vi "Initialize Channel Objects.vi"(8 "error in (no error)":errorcluster, 11 "Default Channel Status":bool) -> (0 "error out":errorcluster, 2 "Active Channel[]":bool[](array[boolean]), 3 "Channel Info[]":T1[](array[typedef]))   [LabVIEW 2020, in "Plugin.lvlib" / "Plugin_UI.lvclass"]
doc: "Creates the default channels."
uses:
  Plugin_UI.lvclass
  builds/Libraries/LabSys Framework.lvlibp/Configuration Storage/Test Configuration/Channel Information.ctl
  builds/Libraries/LabSys Framework.lvlibp/Configuration Storage/Test Configuration/Channel Directions.ctl
  builds/Libraries/LabSys Framework.lvlibp/Configuration Storage/Test Configuration/Scaling Information.ctl
  builds/Libraries/LabSys Framework.lvlibp/Configuration Storage/Test Configuration/Scaling Types.ctl
  builds/Libraries/Framework Base Library.lvlibp/Value Types.ctl
  builds/Libraries/LabSys Framework.lvlibp/Configuration Storage/Test Configuration/Subchannel Information.ctl
  Channels/Output Channels/Output Channels.lvclass
  C:/SVN_LabSys/labsys_lvcode/LabSys_SourceCode/Plugin Template/Source/Code/Channels/Plugin_Channels.lvclass
  Channels/Typedefs/Channel Type.ctl
  Channels/Input Channels/Input Channels.lvclass
  Channels/Plugin_Channels.lvclass
  builds/Libraries/LabSys Framework.lvlibp/Configuration Storage/Test Configuration/Test Configuration.lvclass
  builds/Libraries/Framework Base Library.lvlibp
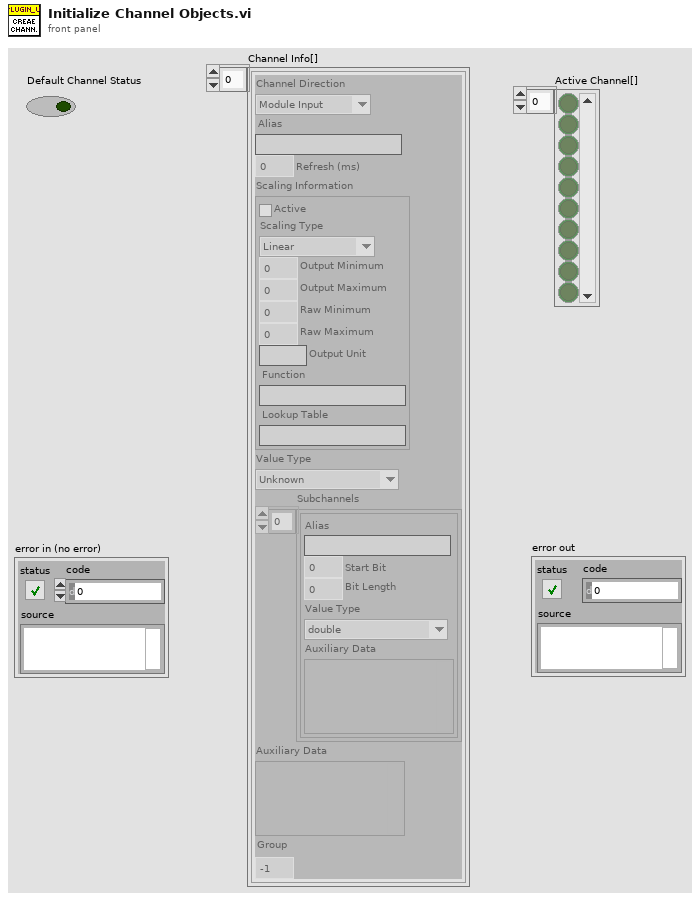
[diagram p1: front panel]
types:
  T1 = typedef "LabSys Framework.lvlibp/Configuration Storage.lvlib/Test Configuration.lvclass/Channel Information.ctl" = cluster{"Channel Direction":T2, "Alias":string, "Refresh (ms)":dbl, "Scaling Information":T3, "Value Type":T5, "Subchannels":T6[], "Auxiliary Data":variant, "Group":i32}
  T2 = typedef "LabSys Framework.lvlibp/Configuration Storage.lvlib/Test Configuration.lvclass/Channel Directions.ctl" = enum8{"Module Input", "Module Output"}
  T3 = typedef "LabSys Framework.lvlibp/Configuration Storage.lvlib/Test Configuration.lvclass/Scaling Information.ctl" = cluster{"Active":bool, "Scaling Type":T4, "Output Minimum":dbl, "Output Maximum":dbl, "Raw Minimum":dbl, "Raw Maximum":dbl, "Output Unit":string, "Function":string, "Lookup Table":string}
  T4 = typedef "LabSys Framework.lvlibp/Configuration Storage.lvlib/Test Configuration.lvclass/Scaling Types.ctl" = enum8{"Linear", "Function", "Lookup Table"}
  T5 = typedef "Framework Base Library.lvlibp/Value Types.ctl" = enum8{"Unknown", "double", "double array", "Waveform", "DigWaveform", "Boolean", "Decimal", "String", "Db2Message", "Byte Array", "Unsigned Decimal"}
  T6 = typedef "LabSys Framework.lvlibp/Configuration Storage.lvlib/Test Configuration.lvclass/Subchannel Information.ctl" = cluster{"Alias":string, "Start Bit":u32, "Bit Length":u32, "Value Type":T5, "Auxiliary Data":variant}
  T7 = typedef "Plugin.lvlib/Plugin_Channels.lvclass/Channel Type.ctl" = enum16{"Input", "Output"}
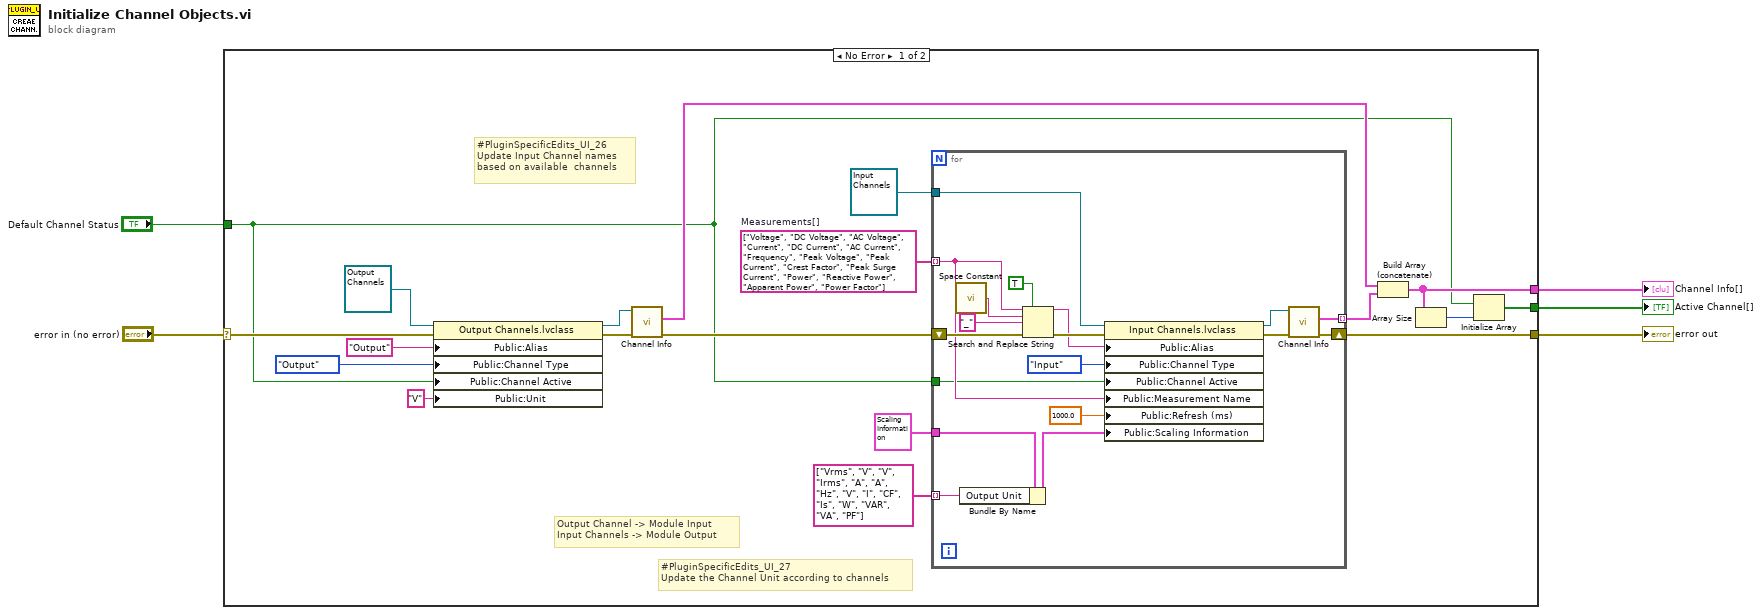
[diagram p0: block diagram]
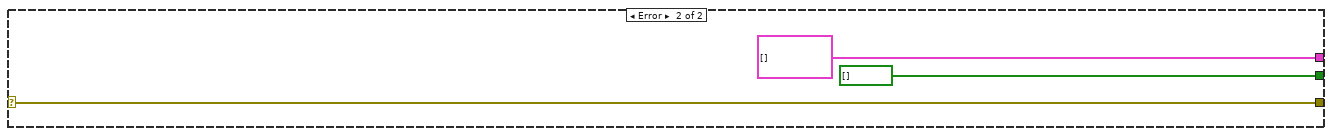
[diagram p2: hidden frame]
diagram:
  n1 = case shown="No Error" "error in (no error)" {
    selector: "error in (no error)" -> [w9 w45]
    tunnel: [w24 bool[] []] -> w5
    tunnel: [w22 T1[] []] -> w4
    tunnel: [w18 w45] -> w3
    tunnel: "Default Channel Status" -> [w8 _]
    frame No Error {
      w16 = string[] ["Voltage", "DC Voltage", "AC Voltage", "Current", "DC Current", "AC Current", "Frequency", "Peak Voltage", "Peak Current", "Crest Factor", "Peak Surge Current", "Power", "Reactive Power", "Apparent Power", "Power Factor"]  # Measurements[]
      # "#PluginSpecificEdits_UI_27 \nUpdate the Channel Unit according to channels"
      # "#PluginSpecificEdits_UI_26\nUpdate Input Channel names \nbased on available  channels"
      # "Output Channel -> Module Input\nInput Channels -> Module Output"
      n2 = property class="Output Channels.lvclass"(reference=refnum<class "Output Channels.lvclass"> refnum ("Plugin.lvlib:Output Channels.lvclass"), error in=w9, "Public:Alias"="Output" ("Alias"), "Public:Channel Type"=Channel_Type."Output" ("Channel Type"), "Public:Channel Active"=w8, "Public:Unit"="V" ("Unit")) -> (reference out=w14:refnum<class "Output Channels.lvclass">, error out=w13:errorcluster)
      n3 = call-dynamic "Channel Info.vi"("error in"=w13, "Output Channels in"=w14) -> ("error out"=w15:errorcluster, "Channel Information"=w19:T1)  [unwired: 6 in, 2 out]
      n4 = for {
        tunnel: refnum<class "Input Channels.lvclass"> refnum ("Plugin.lvlib:Input Channels.lvclass") -> [w42]
        tunnel: w16 -> [w26] mode=indexing
        tunnel: T3 {"Active"=FALSE, "Scaling Type"=enum."Linear", "Output Minimum"=0.0, "Output Maximum"=1.0, "Raw Minimum"=0.0, "Raw Maximum"=1.0, "Output Unit"="", "Function"="", "Lookup Table"=""} ("Scaling Information") -> [w30]
        shift-right: [w32] -> w18
        shift-left: w15 -> [w39]
        tunnel: [w31] -> w21 mode=indexing
        tunnel: string[] ["Vrms", "V", "V", "Irms", "A", "A", "Hz", "V", "I", "CF", "Is", "W", "VAR", "VA", "PF"] -> [w28] mode=indexing
        tunnel: w8 -> [w25]
        n5 = call <vilib>:"Space Constant.vi"() -> ("String"=w36:string)
        n6 = Bundle By Name(cluster=w30, "Output Unit"=w28) -> (w29:T3)
        n7 = Search and Replace String(replace all?=TRUE ("replace all? (F)"), input string=w26, search string=w36, replace string="_" ("replace string (\"\")"), error in=w39) -> (result string=w27:string, error out=w38:errorcluster)  [unwired: 3 in, 2 out]
        n8 = property class="Input Channels.lvclass"(reference=w42, error in=w38, "Public:Alias"=w27, "Public:Channel Type"=Channel_Type."Input" ("Channel Type"), "Public:Channel Active"=w25, "Public:Measurement Name"=w26, "Public:Refresh (ms)"=1000.0 ("Refresh (ms)"), "Public:Scaling Information"=w29) -> (reference out=w33:refnum<class "Input Channels.lvclass">, error out=w34:errorcluster)
        n9 = call-dynamic "Channel Info.vi"("error in"=w34, "Input Channels in"=w33) -> ("error out"=w32:errorcluster, "Channel Information"=w31:T1)  [unwired: 6 in, 2 out]
      }
      n10 = Build Array (concatenate)(w19, w21) -> (w22:T1[])
      n11 = Array Size(array=w22) -> (size(s)=w23:i32)
      n12 = Initialize Array(w8, w23) -> (w24:bool[])
    }
    frame Error {
    }
  }
  "Active Channel[]" <- w5
  "Channel Info[]" <- w4
  "error out" <- w3
